vi "Render Satellites.vi"(7 "Renderer":refnum<class "Renderer.lvclass">, 8 "error in (no error)":errorcluster, 10 "Camera":refnum<class "Camera.lvclass">, 11 "Chmmr in":refnum<class "Chmmr.lvclass">) -> (0 "error out":errorcluster)   [LabVIEW 2021, in "Chmmr.lvclass"]
uses:
  Chmmr.lvclass
  Camera/Camera.lvclass
  Renderer/Renderer.lvclass
  Chmmr.lvclass/Chmmr.ctl
  Vector 2D/Vector 2D.lvclass
  Resource Manager/Resource Manager.lvclass
  Element/Element.lvclass
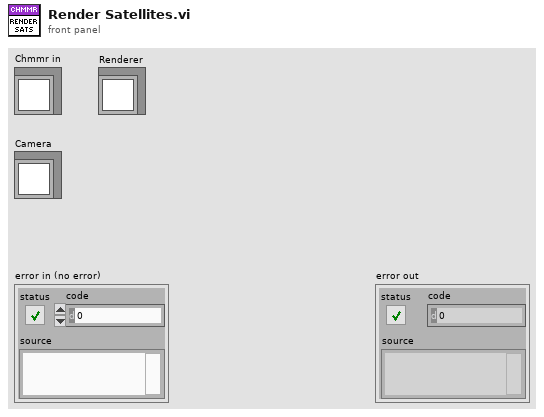
[diagram p1: front panel]
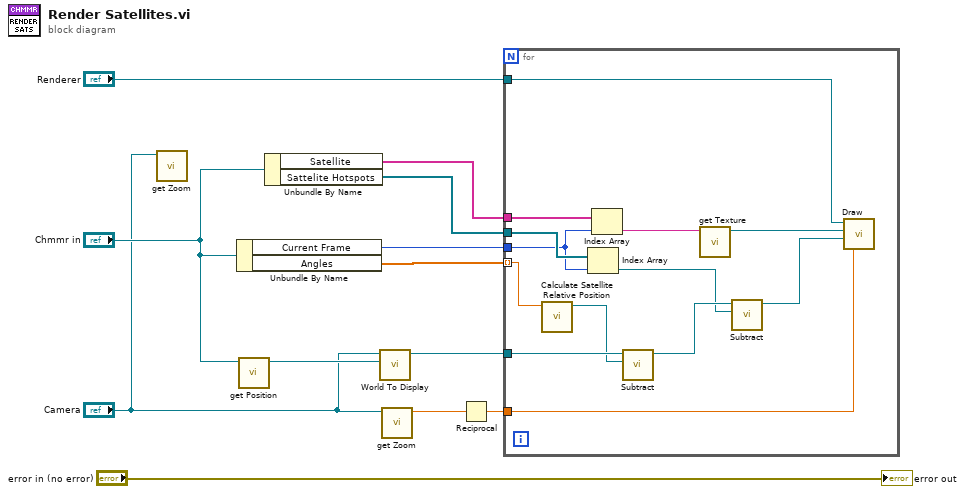
[diagram p0: block diagram]
diagram:
  n1 = call "get Zoom.vi"("Camera in"="Camera") -> ()  [unwired: 10 in, 1 out]
  n2 = Unbundle By Name("Chmmr in") -> ("Current Frame"=w12:i32, "Angles"=w11:sgl[])
  n3 = call "get Position.vi"("Element in"="Chmmr in") -> ("Position"=w4:refnum<class "Vector 2D.lvclass">)  [unwired: 10 in]
  n4 = Unbundle By Name("Chmmr in") -> ("Satellite"=w10:string[], "Sattelite Hotspots"=w9:refnum<class "Vector 2D.lvclass">[])
  n5 = call "World To Display.vi"("World Position"=w4, "Camera in"="Camera") -> ("Display Position"=w7:refnum<class "Vector 2D.lvclass">)  [unwired: 9 in]
  n6 = call "get Zoom.vi"("Camera in"="Camera") -> ("Zoom Level"=w3:sgl)  [unwired: 10 in]
  n7 = Reciprocal(x=w3) -> (1/x=w1:sgl)
  n8 = for {
    tunnel: w9 -> [w23]
    tunnel: w10 -> [w22]
    tunnel: w12 -> [w21]
    tunnel: w11 -> [w20] mode=indexing
    tunnel: w7 -> [w17]
    tunnel: "Renderer" -> [w19]
    tunnel: w1 -> [w18]
    n9 = call "Calculate Satellite Relative Position.vi"("Angle [deg]"=w20) -> ("Position"=w16:refnum<class "Vector 2D.lvclass">)  [unwired: 10 in]
    n10 = Index Array(array=w23, index=w21) -> (element=w14:refnum<class "Vector 2D.lvclass">)
    n11 = Index Array(array=w22, index=w21) -> (element=w25:string)
    n12 = call "Subtract.vi"("B"=w16, "A"=w17) -> ("A-B"=w15:refnum<class "Vector 2D.lvclass">)  [unwired: 9 in]
    n13 = call "get Texture.vi"("Texture Name"=w25) -> ("Texture"=w24:refnum<class "Texture.lvclass">)  [unwired: 10 in]
    n14 = call "Subtract.vi"("B"=w14, "A"=w15) -> ("A-B"=w13:refnum<class "Vector 2D.lvclass">)  [unwired: 9 in]
    n15 = call "Draw.vi"("Scale"=w18, "Destination"=w13, "Texture"=w24, "Renderer"=w19) -> ()  [unwired: 7 in, 1 out]
  }
  "error out" <- "error in (no error)"
